vi "initialize.vi"(7 "VI Refnum":refnum<vi>, 8 "error in":errorcluster, 11 "displayable in":refnum<class "displayable.lvclass">) -> (0 "error out":errorcluster, 3 "displayable":refnum<data-value>)   [LabVIEW 2013, in "displayable.lvclass"]
uses:
  displayable.lvclass
  subscription.ctl
  displayable.lvclass/displayable.ctl
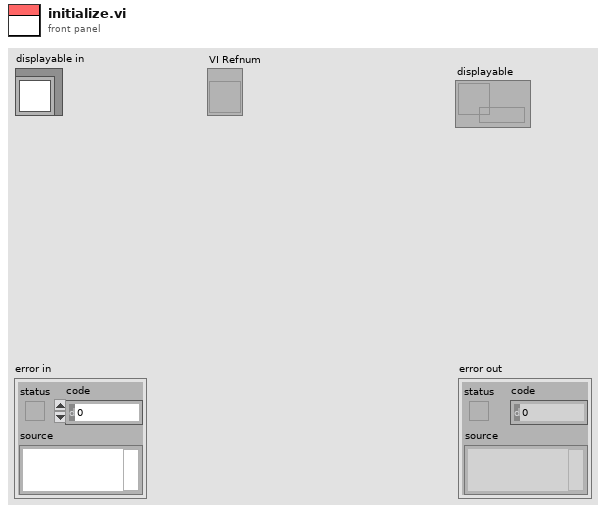
[diagram p1: front panel]
types:
  T1 = typedef "displayable.lvclass/subscription.ctl" = cluster{"control indexes":i32[]}
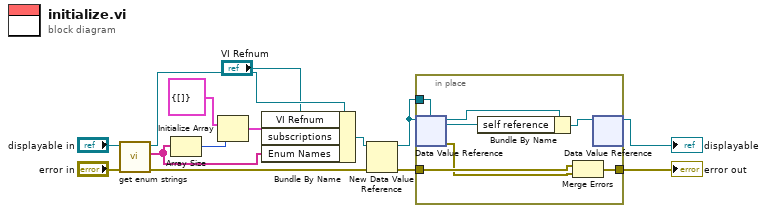
[diagram p0: block diagram]
diagram:
  n1 = call "get enum strings.vi"("error in"="error in", "displayable in"="displayable in") -> ("error out"=w6:errorcluster, "Enum Names"=w11:string[], "displayable out"=w12:refnum<class "displayable.lvclass">)  [unwired: 7 in]
  n2 = Array Size(array=w11) -> (size(s)=w10:i32)
  n3 = Initialize Array(T1 {"control indexes"=[]} ("subscription"), w10) -> (w8:T1[])
  n4 = Bundle By Name(cluster=w12, "VI Refnum"="VI Refnum", "subscriptions"=w8, "Enum Names"=w11) -> (w7:refnum<class "displayable.lvclass">)
  n5 = New Data Value Reference(data value=w7, error in=w6) -> (data value reference=w4:refnum<data-value>, error out=w3:errorcluster)
  n6 = in-place {
    in-place-border: w4 -> [w18]
    in-place-border: w3 -> [w17]
    in-place-border: [w15] -> w2
    n7 = in-place-dvr #1(w4) -> (w20:refnum<class "displayable.lvclass">, w16:errorcluster)
    n8 = Bundle By Name(cluster=w20, "self reference"=w18) -> (w19:refnum<class "displayable.lvclass">)
    n9 = Merge Errors(w17, w16) -> (w15:errorcluster)
    n10 = in-place-dvr #1(w19) -> (→"displayable":refnum<data-value>)  [unwired: 1 out]
  }
  "error out" <- w2
